vi "SetPosition.vi"(8 "error in (no error)":errorcluster, 10 "position":cluster{"left":u32, "top":u32}, 11 "frame in":refnum<class "frame.lvclass">) -> (0 "error out":errorcluster, 3 "frame out":refnum<class "frame.lvclass">)   [LabVIEW 2009, in "frame.lvclass"]
uses:
  frame.lvclass
  frame.lvclass/frame.ctl
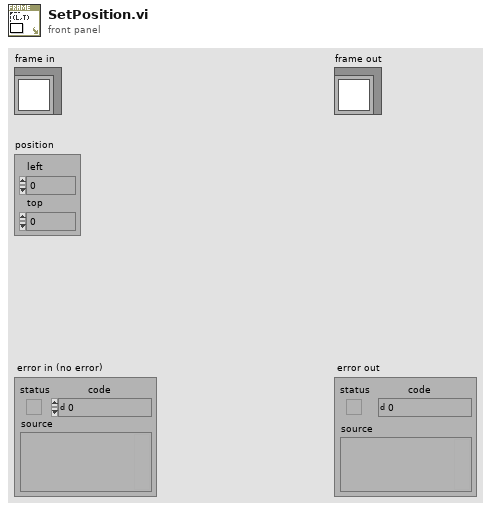
[diagram p1: front panel]
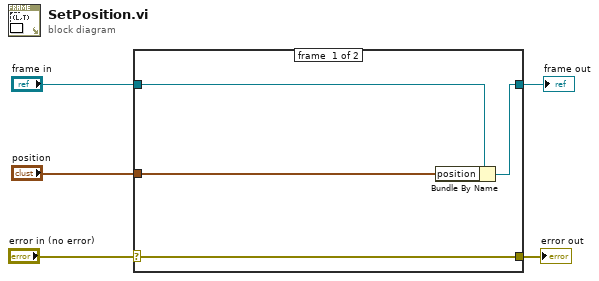
[diagram p0: block diagram]
diagram:
  n1 = case shown="No Error" "error in (no error)" {
    selector: "error in (no error)" -> [w9 w10]
    tunnel: [w9 w10] -> w2
    tunnel: [w7 w11] -> w4
    tunnel: "frame in" -> [w8 w11]
    tunnel: "position" -> [w6 _]
    frame #0 {
      n2 = Bundle By Name(cluster=w8, "position"=w6) -> (w7:refnum<class "frame.lvclass">)
    }
    frame #1 {
    }
  }
  "error out" <- w2
  "frame out" <- w4
